vi "CalibratedGrating.vi"(0 "Grating:":u16(ring) items=["Shimadzu 30-006  "], 1 "Subvi?":bool, 2 "Laser:":u16(ring) items=["800nm  "], 3 "Harmonic":dbl min=10.0 max=40.0, 4 "Caibration Date":u16(ring) items=["first calibration - 7/31", "7/31-current"]) -> (5 "Position on spectrometer (pixels):":dbl)   [LabVIEW 2019]
panel:
  in  "Stop":bool
  out "Highest Harmonic:":dbl
  out "Lowest Harmonic:":dbl
  out "Beta2 (deg):":dbl
  out "Beta1 (deg):":dbl
  out "Anglular position of peak (deg):":dbl
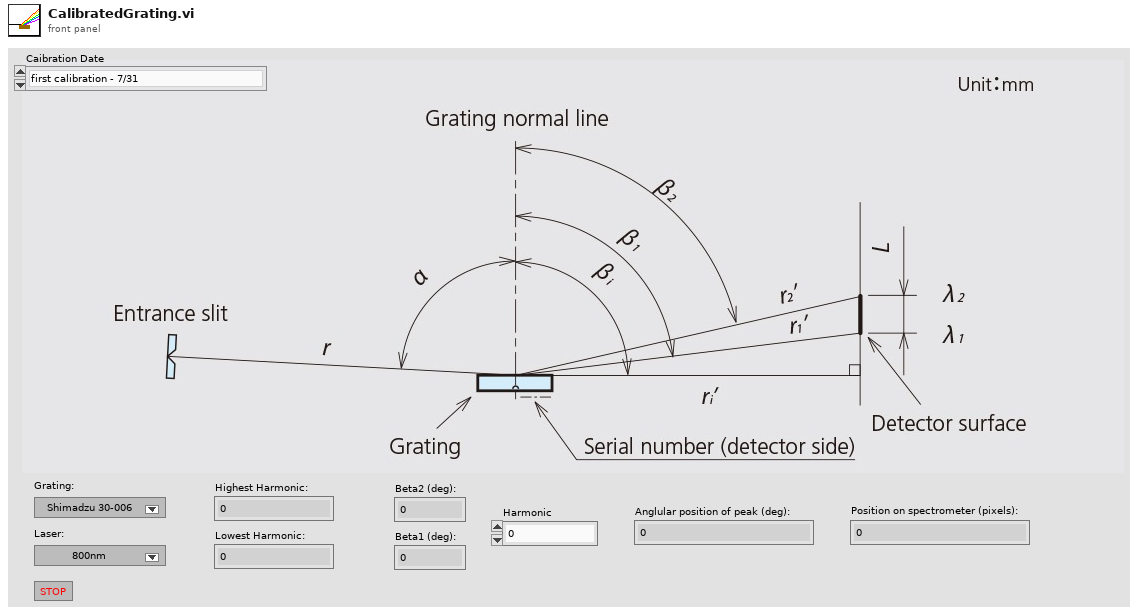
[diagram p1: front panel]
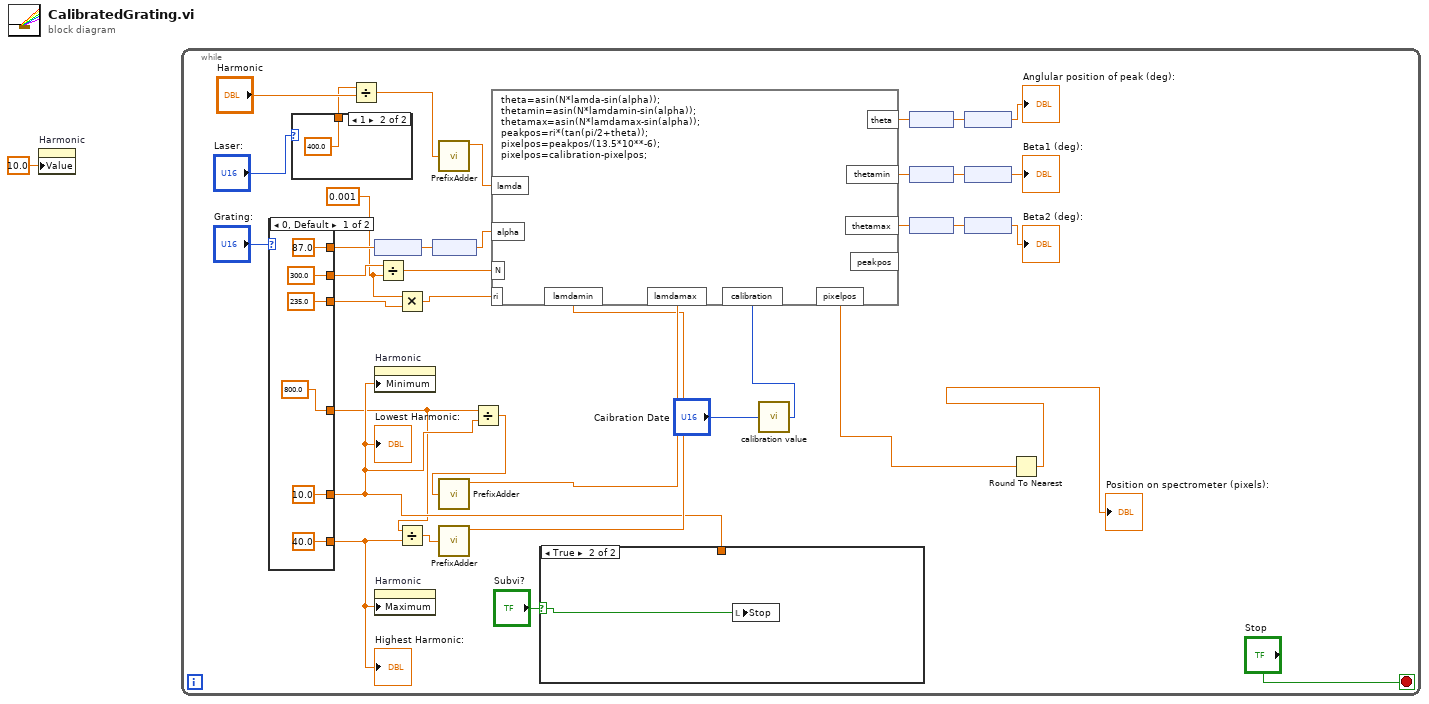
[diagram p0: block diagram]
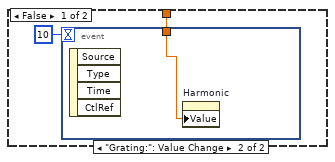
[diagram p2: hidden frame]
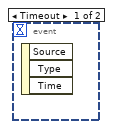
[diagram p3: hidden frame]
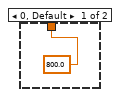
[diagram p4: hidden frame]
diagram:
  n1 = property on="Harmonic" class="DigNum (strict)"("Value"=10.0 ("Wavelegnth (nm)")) -> ()  [unwired: 2 in, 2 out]
  n2 = while {
    stop <- "Stop" stop-if-true
    w18 = 0.001 ("y")
    n3 = case shown="0, Default" "Grating:" {
      tunnel: [300.0 _] -> w34
      tunnel: [87.0 _] -> w33
      tunnel: [10.0 _] -> w9
      tunnel: [40.0 _] -> w10
      tunnel: [235.0 _] -> w20
      tunnel: [800.0 _] -> w7
      frame 0, Default {
      }
      frame 1 {
      }
    }
    "Lowest Harmonic:" <- w9
    "Highest Harmonic:" <- w10
    n4 = case shown="1" "Laser:" {
      tunnel: [800.0 400.0] -> w8
      frame 0, Default {
      }
      frame 1 {
      }
    }
    n5 = Divide(x=w8, y="Harmonic") -> (x/y=w16:dbl)
    n6 = node(w33) -> (w32:dbl[unit])
    n7 = property on="Harmonic" class="DigNum (strict)"("Minimum"=w9) -> ()  [unwired: 2 in, 2 out]
    n8 = property on="Harmonic" class="DigNum (strict)"("Maximum"=w10) -> ()  [unwired: 2 in, 2 out]
    n9 = Divide(x=w34, y=w18) -> (x/y=w35:dbl)
    n10 = Multiply(x=w18, y=w20) -> (x*y=w19:dbl)
    n11 = Divide(x=w7, y=w10) -> (x/y=w12:dbl)
    n12 = node(w32) -> (w31:dbl)
    n13 = call "PrefixAdder.vi"("No prefix"=w16) -> ("Nano"=w36:dbl)  [unwired: 3 out]
    n14 = call "PrefixAdder.vi"("No prefix"=w12) -> ("Nano"=w13:dbl)  [unwired: 3 out]
    n15 = Divide(x=w7, y=w9) -> (x/y=w11:dbl)
    n16 = call "PrefixAdder.vi"("No prefix"=w11) -> ("Nano"=w14:dbl)  [unwired: 3 out]
    n17 = case shown="True" "Subvi?" {
      selector: "Subvi?" -> [_ w41]
      tunnel: w9 -> [w38 _]
      frame False {
        n18 = event shown="[1] \"Grating:\": Value Change" {
          selector: _ -> [_ _]
          dyn-events: _ -> [_ _]
          timeout: 10 -> [_ _]
          tunnel: w38 -> [_ w40]
          event Timeout {
            n19 = event-data() -> ()  [unwired: 1 in, 3 out]
          }
          event "Grating:": Value Change {
            n20 = event-data() -> ()  [unwired: 1 in, 4 out]
            n21 = property on="Harmonic" class="DigNum (strict)"("Value"=w40) -> ()  [unwired: 2 in, 2 out]
          }
        }
      }
      frame True {
        n22 = local write "Stop"(w41) -> ()
      }
    }
    n23 = call "calibration value.vi"("Caibration Date"="Caibration Date") -> ("Numeric"=w3:i32)
    n24 = formula code="theta=asin(N*lamda-sin(alpha));\nthetamin=asin(N*lamdamin-sin(alpha));\nthetamax=asin(N*lamdamax-sin(alpha));\npeakpos=ri*(tan(pi/2+theta));\npixelpos=peakpos/(13.5*10**-6);\npixelpos=calibration-pixelpos;"("lamda"=w36, "N"=w35, "alpha"=w31, "lamdamin"=w13, "lamdamax"=w14, "ri"=w19, "calibration"=w3) -> ("theta"=w21:dbl, "thetamin"=w25:dbl, "thetamax"=w26:dbl, "pixelpos"=w5:dbl)  [unwired: 1 out]
    n25 = node(w21) -> (w30:dbl[unit])
    n26 = node(w25) -> (w28:dbl[unit])
    n27 = node(w26) -> (w27:dbl[unit])
    n28 = node(w30) -> (→"Anglular position of peak (deg):":dbl)
    n29 = node(w28) -> (→"Beta1 (deg):":dbl)
    n30 = node(w27) -> (→"Beta2 (deg):":dbl)
    n31 = Round To Nearest(number=w5) -> (nearest integer value=→"Position on spectrometer (pixels):":dbl)
  }
